vi "QcmDemo.vi"() -> ()   [LabVIEW 2012]
panel:
  out "FitTime":dbl
  out "FitChiSquared":dbl
  out "FitAcceptable":bool
  out "AcquisitionTime":dbl
  out "Calibration Factor":dbl=226.0 format="%.3f"
  out "Area of Overlap":dbl=0.205 format="%#.6f"
  out "Freq. Step":dbl=0.2 format="%.3f"
  out "Spectrum":cluster{ext[], ext[]}[](graph)
  in  "TEST":bool
  out "ScanError":bool
  in  "stop":bool
  out "Data Done":bool
  out "Data Available":bool
  out "fp":dbl format="%_8f"
  out "fs":dbl format="%_8f"
  out "Amplitude":i16(slide)=50 min=1 max=100 step=1 scale=0.0..100.0
  out "DampingLevel":i16=1
  out "Freq. Width":dbl=65537.373 format="%^#.6e"
  out "Center Freq.":dbl=9992621.0
  out "SerialNo":string
  in  "GAMRYCOMLib.IGamryQcm":refnum<k7>
  out "fs and fp":cluster{"fs":dbl, "fp":dbl}(graph)={"fs"=9.9831777135, "fp"=10.0088607135}
  out "error out":errorcluster
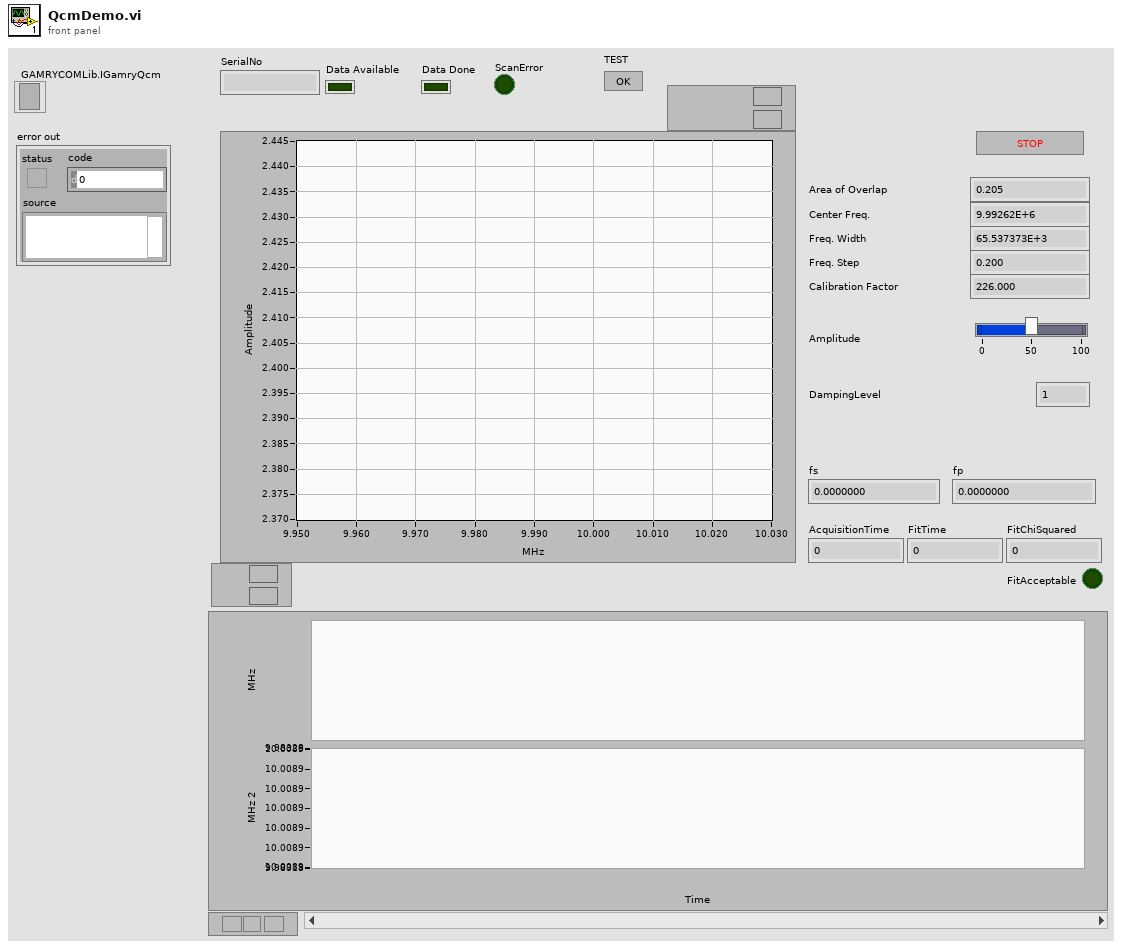
[diagram p1: front panel]
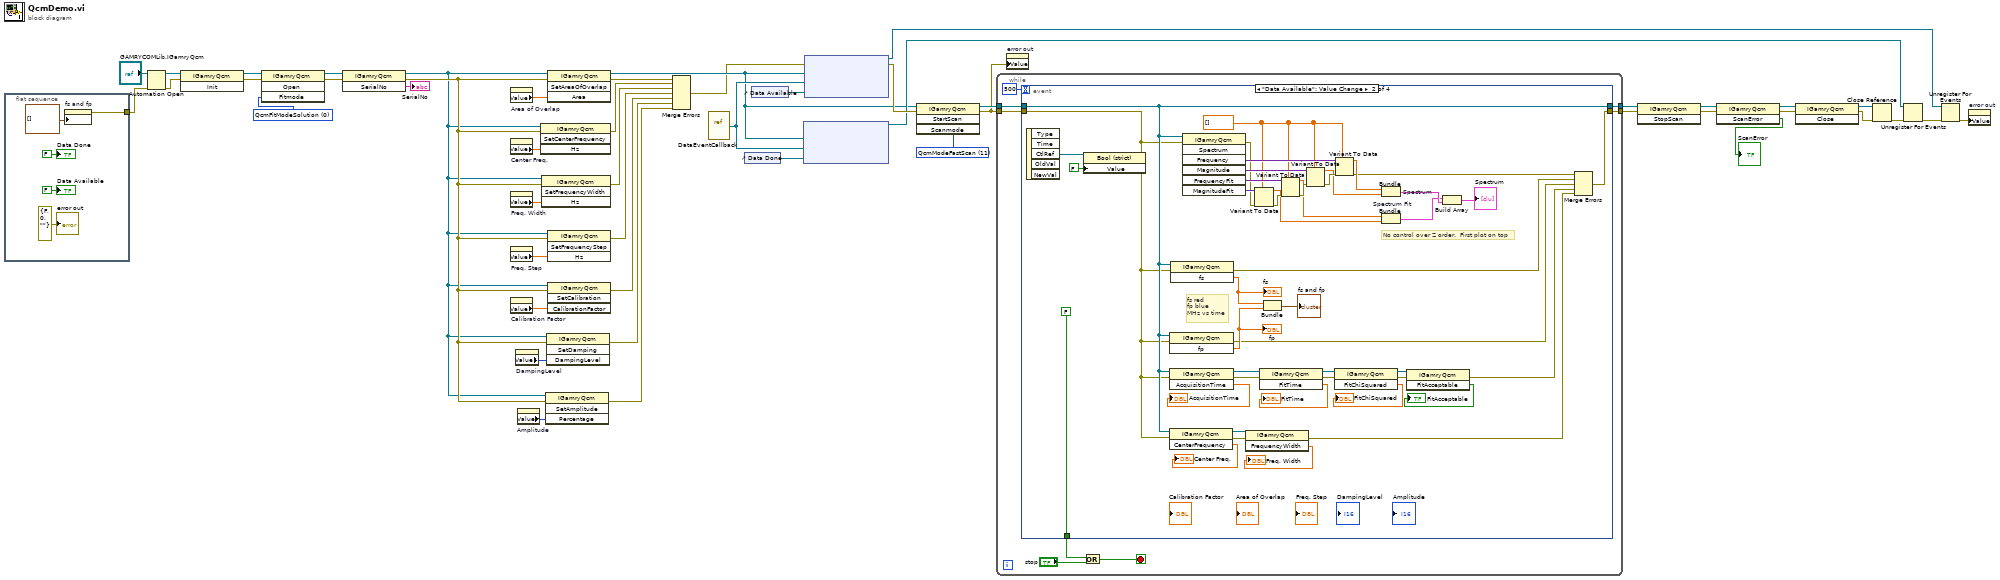
[diagram p0: block diagram]
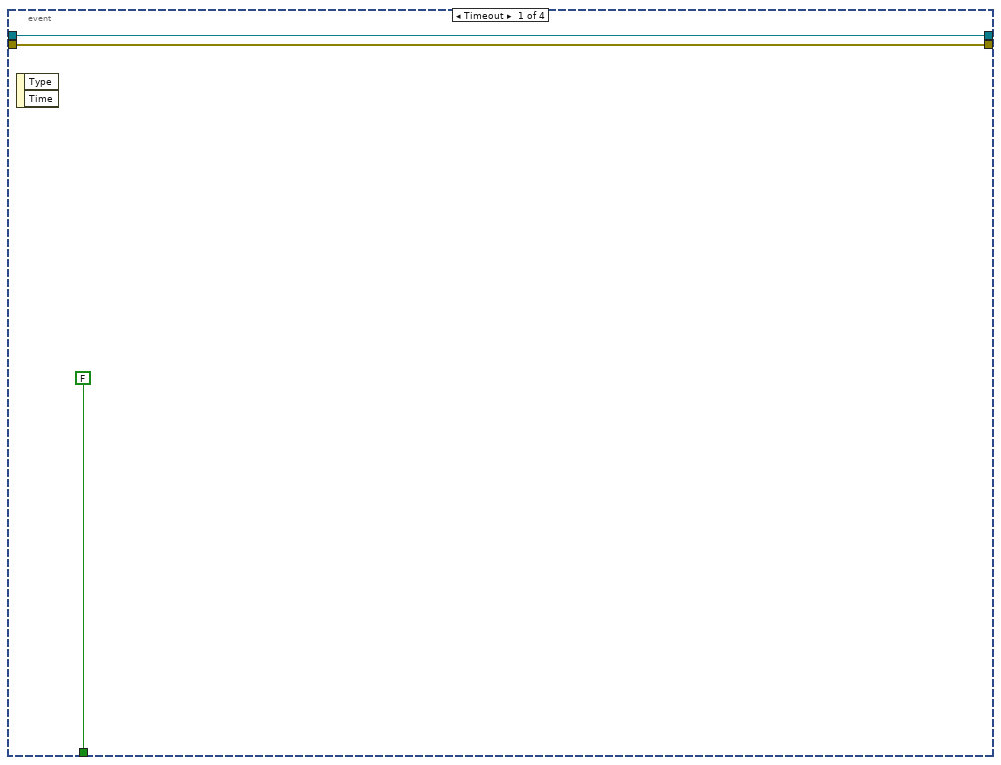
[diagram p2: hidden frame]
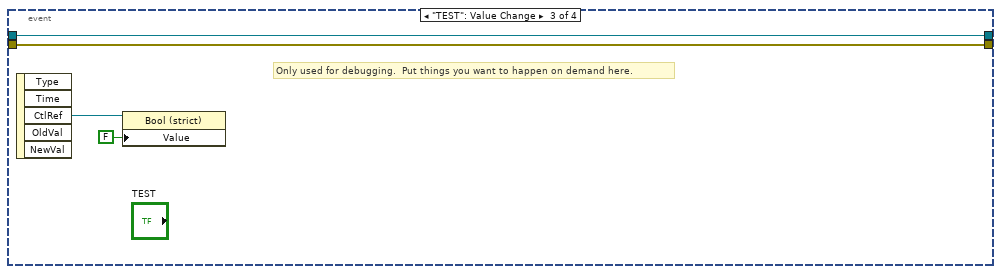
[diagram p3: hidden frame]
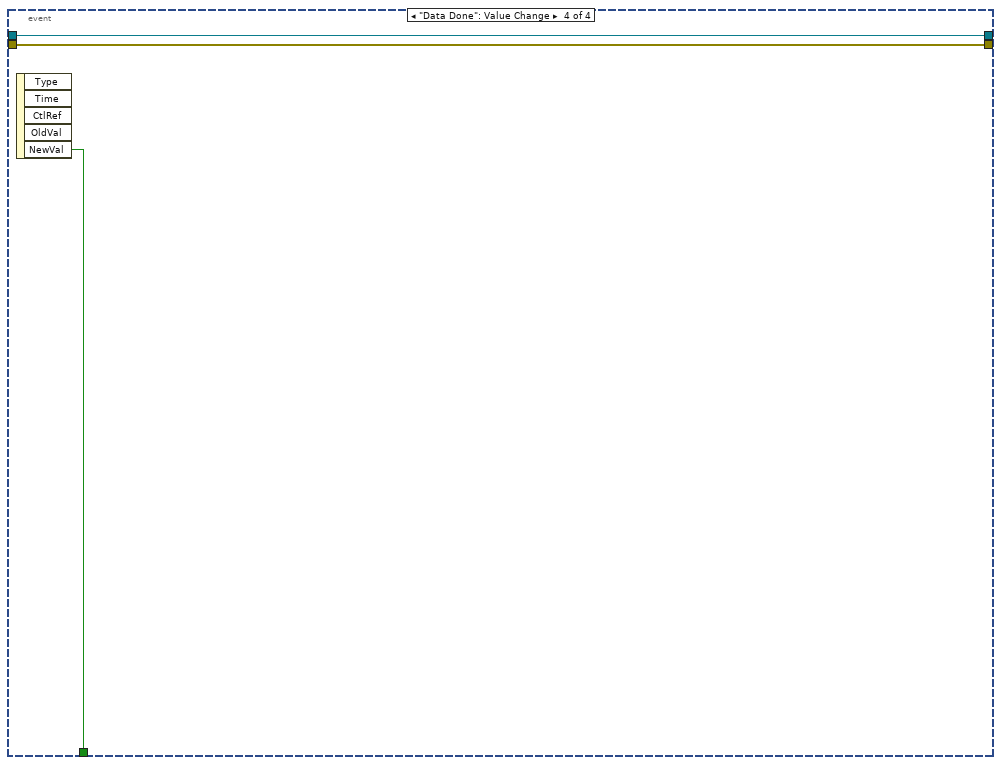
[diagram p4: hidden frame]
diagram:
  w40 = 11 items=["QcmModeIdle"=0, "QcmModeFastScan"=11, "QcmModeSingleScan"=12] ("Scanmode")
  w44 = 0 items=["QcmFitModeSolution", "QcmFitModeAir"] ("Fitmode")
  n1 = flat-sequence {
    tunnel: [w51] -> w31
    frame #0 {
      n2 = property on="fs and fp" class="WFChart (strict)"("History Data"=cluster{"fs":dbl, "fp":dbl}[] []) -> (error out=w51:errorcluster)  [unwired: 2 in, 1 out]
      "error out" <- errorcluster {"status"=FALSE, "code"=0, "source"=""} ("error out")
      "Data Done" <- FALSE ("Data Done")
      "Data Available" <- FALSE ("Data Available")
    }
  }
  n3 = Automation Open(error in (no error)=w31, Automation Refnum="GAMRYCOMLib.IGamryQcm") -> (Automation Refnum=w48:refnum<k7>, error out=w47:errorcluster)  [unwired: 2 in]
  n4 = invoke class="IGamryQcm" method="Init"(reference=w48, error in=w47) -> (reference out=w46:refnum<k7>, error out=w45:errorcluster)  [unwired: 1 in, 1 out]
  n5 = invoke class="IGamryQcm" method="Open"(reference=w46, error in=w45, "Fitmode"=w44) -> (reference out=w43:refnum<k7>, error out=w42:errorcluster)  [unwired: 1 in, 2 out]
  n6 = invoke class="IGamryQcm" method="SerialNo"(reference=w43, error in=w42) -> (reference out=w1:refnum<k7>, error out=w2:errorcluster, "SerialNo"=→"SerialNo":string)  [unwired: 1 in]
  n7 = property on="Area of Overlap" class="DigNum (strict)"() -> ("Value"=w15:dbl)  [unwired: 2 in, 2 out]
  n8 = property on="Center Freq." class="DigNum (strict)"() -> ("Value"=w18:dbl)  [unwired: 2 in, 2 out]
  n9 = property on="Freq. Width" class="DigNum (strict)"() -> ("Value"=w17:dbl)  [unwired: 2 in, 2 out]
  n10 = property on="Freq. Step" class="DigNum (strict)"() -> ("Value"=w16:dbl)  [unwired: 2 in, 2 out]
  n11 = property on="Calibration Factor" class="DigNum (strict)"() -> ("Value"=w14:dbl)  [unwired: 2 in, 2 out]
  n12 = property on="DampingLevel" class="DigNum (strict)"() -> ("Value"=w13:i16)  [unwired: 2 in, 2 out]
  n13 = property on="Amplitude" class="Slide (strict)"() -> ("Value"=w12:i16)  [unwired: 2 in, 2 out]
  n14 = invoke class="IGamryQcm" method="SetCenterFrequency"(reference=w1, error in=w2, "Hz"=w18) -> (error out=w10:errorcluster)  [unwired: 1 in, 3 out]
  n15 = invoke class="IGamryQcm" method="SetFrequencyWidth"(reference=w1, error in=w2, "Hz"=w17) -> (error out=w9:errorcluster)  [unwired: 1 in, 3 out]
  n16 = invoke class="IGamryQcm" method="SetAmplitude"(reference=w1, error in=w2, "Percentage"=w12) -> (error out=w3:errorcluster)  [unwired: 1 in, 3 out]
  n17 = invoke class="IGamryQcm" method="SetDamping"(reference=w1, error in=w2, "DampingLevel"=w13) -> (error out=w6:errorcluster)  [unwired: 1 in, 3 out]
  n18 = invoke class="IGamryQcm" method="SetAreaOfOverlap"(reference=w1, error in=w2, "Area"=w15) -> (reference out=w5:refnum<k7>, error out=w11:errorcluster)  [unwired: 1 in, 2 out]
  n19 = invoke class="IGamryQcm" method="SetFrequencyStep"(reference=w1, error in=w2, "Hz"=w16) -> (error out=w8:errorcluster)  [unwired: 1 in, 3 out]
  n20 = invoke class="IGamryQcm" method="SetCalibration"(reference=w1, error in=w2, "CalibrationFactor"=w14) -> (error out=w7:errorcluster)  [unwired: 1 in, 3 out]
  n21 = Merge Errors(w11, w10, w9, w8, w7, w6, w3) -> (w4:errorcluster)
  n22 = vi-ref "DataEventCallback.vi"() -> ("vi reference"=w36:refnum<vi>)
  n23 = control-ref of="Data Done"() -> (w38:refnum<vi>)
  n24 = control-ref of="Data Available"() -> (w37:refnum<vi>)
  n25 = node(w5, w36, w38) -> (w22:refnum<k27>)  [unwired: 2 in, 1 out]
  n26 = node(w4, w5, w36, w37) -> (w23:refnum<k27>, w39:errorcluster)  [unwired: 1 in]
  n27 = invoke class="IGamryQcm" method="StartScan"(reference=w5, error in=w39, "Scanmode"=w40) -> (reference out=w35:refnum<k7>, error out=w34:errorcluster)  [unwired: 1 in, 2 out]
  n28 = while {
    tunnel: w35 -> [w62]
    tunnel: w34 -> [w61]
    tunnel: [w57] -> w33
    tunnel: [w56] -> w32
    stop <- w58 stop-if-true
    n29 = event shown="[1] \"Data Available\": Value Change" {
      selector: _ -> [_ _ _ _]
      dyn-events: _ -> [_ _ _ _]
      timeout: 500 -> [_ _ _ _]
      tunnel: w61 -> [w64 w67 w110 w115]
      tunnel: w62 -> [w65 w68 w111 w116]
      tunnel: [w65 w68 w111 w116] -> w57
      tunnel: [w64 w105 w110 w115] -> w56
      tunnel: [FALSE ("NewVal") FALSE ("NewVal") _ w114] -> w60
      event Timeout {
        n30 = event-data() -> ()  [unwired: 1 in, 2 out]
      }
      event "Data Available": Value Change {
        w95 = ext[] []
        # "No control over Z order.  First plot on top"
        # "fs red\nfp blue\nMHz vs time"
        n31 = event-data() -> ("CtlRef"=w109:refnum<vi>)  [unwired: 1 in, 4 out]
        n32 = property class="Bool (strict)"(reference=w109, "Value"=FALSE) -> ()  [unwired: 1 in, 2 out]
        n33 = invoke class="IGamryQcm" method="CenterFrequency"(reference=w68, error in=w67) -> (reference out=w69:refnum<k7>, error out=w70:errorcluster, "CenterFrequency"=→"Center Freq.":dbl)  [unwired: 1 in]
        n34 = invoke class="IGamryQcm" method="fp"(reference=w68, error in=w67) -> (error out=w81:errorcluster, "fp"=w106:dbl)  [unwired: 1 in, 1 out]
        "fp" <- w106
        n35 = invoke class="IGamryQcm" method="AcquisitionTime"(reference=w68, error in=w67) -> (reference out=w77:refnum<k7>, error out=w76:errorcluster, "AcquisitionTime"=→"AcquisitionTime":dbl)  [unwired: 1 in]
        n36 = invoke class="IGamryQcm" method="fs"(reference=w68, error in=w67) -> (error out=w82:errorcluster, "fs"=w107:dbl)  [unwired: 1 in, 1 out]
        "fs" <- w107
        n37 = invoke class="IGamryQcm" method="Spectrum"(reference=w68, error in=w67) -> (error out=w99:errorcluster, "Frequency"=w103:variant, "Magnitude"=w102:variant, "FrequencyFit"=w101:variant, "MagnitudeFit"=w100:variant)  [unwired: 5 in, 2 out]
        n38 = invoke class="IGamryQcm" method="FrequencyWidth"(reference=w69, error in=w70) -> (error out=w66:errorcluster, "FrequencyWidth"=→"Freq. Width":dbl)  [unwired: 1 in, 1 out]
        n39 = Variant To Data(error in=w99, type=w95, Variant=w100) -> (data=w90:ext[], error out=w98:errorcluster)
        n40 = invoke class="IGamryQcm" method="FitTime"(reference=w77, error in=w76) -> (reference out=w75:refnum<k7>, error out=w74:errorcluster, "FitTime"=→"FitTime":dbl)  [unwired: 1 in]
        n41 = Bundle("fs"=w107, "fp"=w106) -> (→"fs and fp":cluster{"fs":dbl, "fp":dbl})  [unwired: 1 in]
        n42 = Variant To Data(error in=w98, type=w95, Variant=w101) -> (data=w91:ext[], error out=w97:errorcluster)
        n43 = Variant To Data(error in=w97, type=w95, Variant=w102) -> (data=w93:ext[], error out=w96:errorcluster)
        n44 = invoke class="IGamryQcm" method="FitChiSquared"(reference=w75, error in=w74) -> (reference out=w80:refnum<k7>, error out=w79:errorcluster, "FitChiSquared"=→"FitChiSquared":dbl)  [unwired: 1 in]
        n45 = Variant To Data(error in=w96, type=w95, Variant=w103) -> (data=w94:ext[], error out=w83:errorcluster)
        n46 = Bundle "Spectrum"(w94, w93) -> (w89:cluster{ext[], ext[]})  [unwired: 1 in]
        n47 = Bundle "Spectrum Fit"(w91, w90) -> (w88:cluster{ext[], ext[]})  [unwired: 1 in]
        n48 = invoke class="IGamryQcm" method="FitAcceptable"(reference=w80, error in=w79) -> (error out=w78:errorcluster, "FitAcceptable"=→"FitAcceptable":bool)  [unwired: 1 in, 1 out]
        n49 = Build Array(w88, w89) -> (→"Spectrum":cluster{ext[], ext[]}[])
        n50 = Merge Errors(w83, w82, w81, w78, w66) -> (w105:errorcluster)
      }
      event "TEST": Value Change {
        # "Only used for debugging.  Put things you want to happen on demand here."
        n51 = event-data() -> ("CtlRef"=w113:refnum<vi>)  [unwired: 1 in, 4 out]
        n52 = property class="Bool (strict)"(reference=w113, "Value"=FALSE) -> ()  [unwired: 1 in, 2 out]
      }
      event "Data Done": Value Change {
        n53 = event-data() -> ("NewVal"=w114:bool)  [unwired: 1 in, 4 out]
      }
    }
    n54 = Or(x=w60, y="stop") -> (x .or. y?=w58:bool)
  }
  n55 = property on="error out" class="Clust (strict)"("Value"=w34) -> ()  [unwired: 2 in, 2 out]
  n56 = invoke class="IGamryQcm" method="StopScan"(reference=w33, error in=w32) -> (reference out=w30:refnum<k7>, error out=w29:errorcluster)  [unwired: 1 in, 1 out]
  n57 = invoke class="IGamryQcm" method="ScanError"(reference=w30, error in=w29) -> (reference out=w28:refnum<k7>, error out=w27:errorcluster, "ScanError"=→"ScanError":bool)  [unwired: 1 in]
  n58 = invoke class="IGamryQcm" method="Close"(reference=w28, error in=w27) -> (reference out=w24:refnum<k7>, error out=w25:errorcluster)  [unwired: 1 in, 1 out]
  n59 = Close Reference(reference=w24, error in (no error)=w25) -> (error out=w21:errorcluster)
  n60 = Unregister For Events(event registration refnum=w22, error in=w21) -> (error out=w20:errorcluster)
  n61 = Unregister For Events(event registration refnum=w23, error in=w20) -> (error out=w19:errorcluster)
  n62 = property on="error out" class="Clust (strict)"("Value"=w19) -> ()  [unwired: 2 in, 2 out]
